vi "TTA_MATLAB_Set_Channels.vi"(8 "error in":errorcluster, 10 "Tile Section":enum16{"RFIC", "TX", "RX"}(ring), 11 "Channel Cluster":cluster{"Channel 1":bool, "Channel 2":bool}) -> (0 "error out":errorcluster)   [LabVIEW 2016]
uses:
  TTA_Globals/Test_Environment.vi
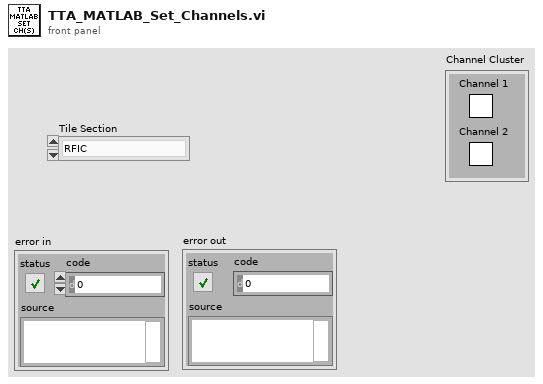
[diagram p1: front panel]
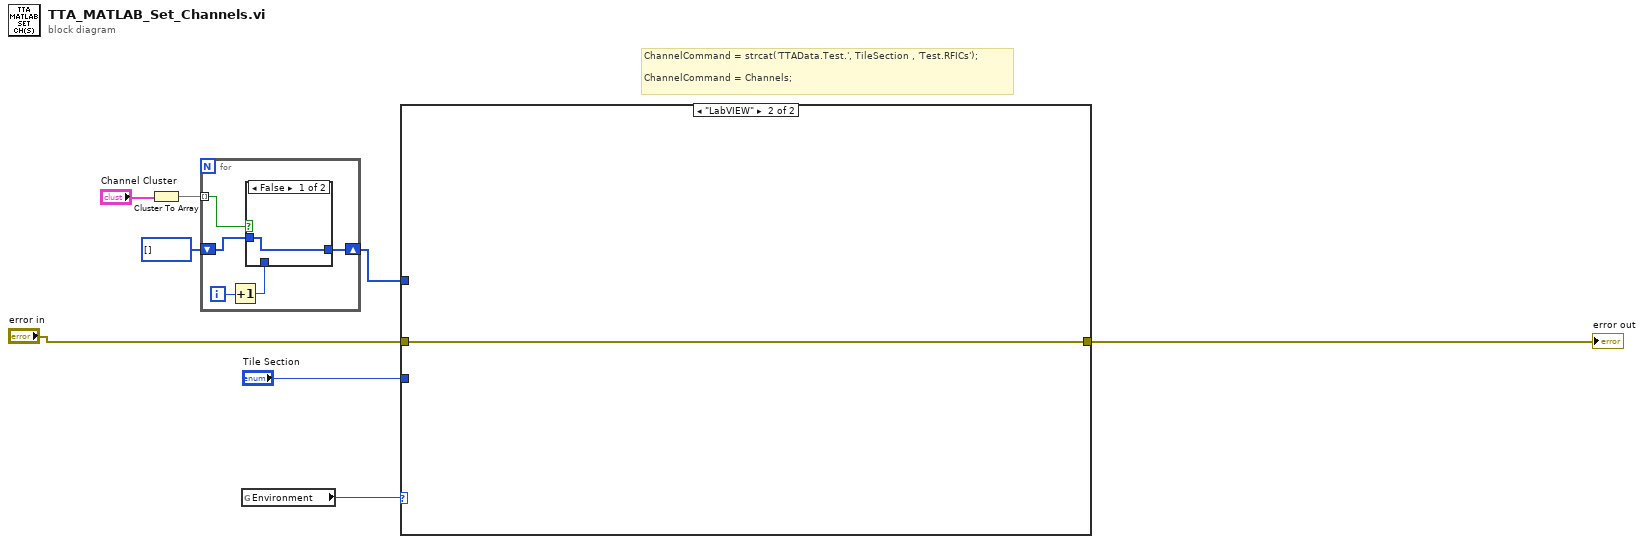
[diagram p0: block diagram]
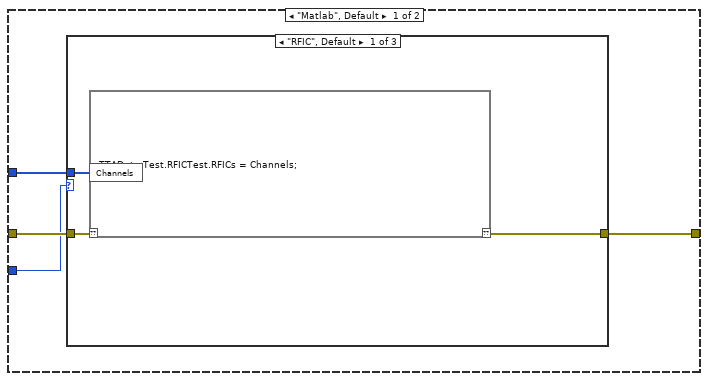
[diagram p2: hidden frame]
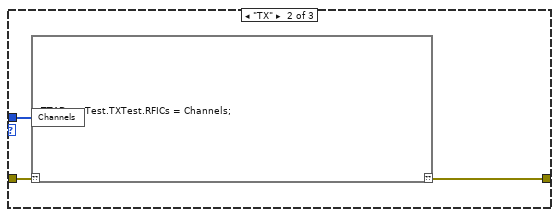
[diagram p3: hidden frame]
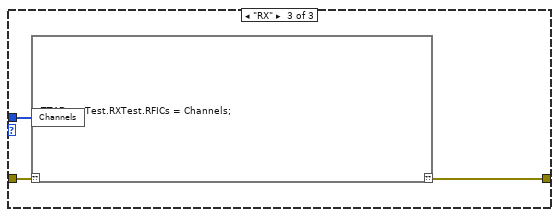
[diagram p4: hidden frame]
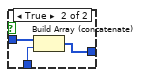
[diagram p5: hidden frame]
diagram:
  # "ChannelCommand = strcat('TTAData.Test.', TileSection , 'Test.RFICs');\n\nChannelCommand = Channels;"
  n1 = Cluster To Array(cluster="Channel Cluster") -> (array=w6:bool[])
  n2 = for {
    tunnel: w6 -> [w13] mode=indexing
    shift-right: [w10] -> w3
    shift-left: i32[] [] -> [w9]
    i -> [w12]
    n3 = Increment(x=w12) -> (x+1=w11:i32)
    n4 = case shown="False" w13 {
      tunnel: w11 -> [_ w17]
      tunnel: [w14 w16] -> w10
      tunnel: w9 -> [w14 w15]
      frame False {
      }
      frame True {
        n5 = Build Array (concatenate)(w15, w17) -> (w16:i32[])
      }
    }
  }
  n6 = global read "Test_Environment.vi" "Environment"() -> (w1:enum16{"Matlab", "LabVIEW"})
  n7 = case shown="\"LabVIEW\"" w1 {
    tunnel: [w21 w31] -> w8
    tunnel: "error in" -> [w20 w31]
    tunnel: w3 -> [w19 _]
    tunnel: "Tile Section" -> [w18 _]
    frame "Matlab", Default {
      n8 = case shown="\"RFIC\", Default" w18 {
        tunnel: [w24 w27 w30] -> w21
        tunnel: w20 -> [w23 w26 w29]
        tunnel: w19 -> [w22 w25 w28]
        frame "RFIC", Default {
          n9 = script code="TTAData.Test.RFICTest.RFICs = Channels;"("??"=w23, "Channels"=w22) -> ("??"=w24:errorcluster)
        }
        frame "TX" {
          n10 = script code="TTAData.Test.TXTest.RFICs = Channels;"("??"=w26, "Channels"=w25) -> ("??"=w27:errorcluster)
        }
        frame "RX" {
          n11 = script code="TTAData.Test.RXTest.RFICs = Channels;"("??"=w29, "Channels"=w28) -> ("??"=w30:errorcluster)
        }
      }
    }
    frame "LabVIEW" {
    }
  }
  "error out" <- w8
